vi "setAutoMinMax.vi"(0 "Camera in":refnum<class "Camera.lvclass">, 5 "data_format":T1(ring)=enum."Mono16", 7 "image":u16[][](array[numeric]), 11 "error in (no error)":errorcluster) -> (4 "Camera out":refnum<class "Camera.lvclass">, 15 "error out":errorcluster)   [LabVIEW 2019, in "Camera.lvclass"]
doc: "Retreive the rec handle.\nThis handle allows direct access to all underlying functions of the pco.recorder."
uses:
  Camera.lvclass
  pco.convert/Convert.lvlib
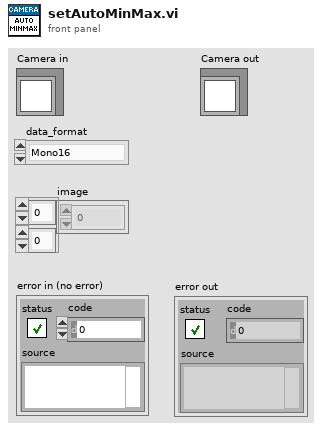
[diagram p1: front panel]
types:
  T1 = enum16{"Undefined", "Mono8", "Mono16", "BGRA8", "RGBA8", "BGRA16", "RGBA16", "CompressedMono8"}
  T2 = cluster{"wScale_minmax":u16, "iScale_maxmax":i32, "iScale_min":i32, "iScale_max":i32, "iColor_temp":i32, "iColor_tint":i32, "iColor_saturation":i32, "iColor_vibrance":i32, "iContrast":i32, "iGamma":i32, "iSRGB":i32, "pHistogramData":u64, "dwProcessingFlags":u32, "wProzValue4Min":u16, "wProzValue4Max":u16}
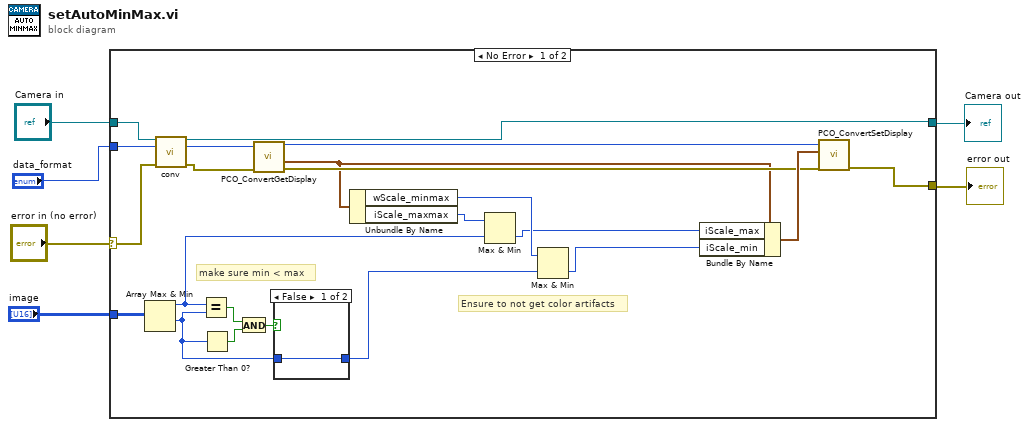
[diagram p0: block diagram]
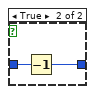
[diagram p2: hidden frame]
diagram:
  n1 = case shown="No Error" "error in (no error)" {
    selector: "error in (no error)" -> [w27 w33]
    tunnel: [w15 w33] -> w4
    tunnel: [w16 w32] -> w5
    tunnel: "Camera in" -> [w28 w32]
    tunnel: "image" -> [w24 _]
    tunnel: "data_format" -> [w14 _]
    frame No Error {
      # "Ensure to not get color artifacts"
      # "make sure min < max"
      n2 = Array Max & Min(array=w24) -> (max value=w12:u16, min value=w20:u16)  [unwired: 2 out]
      n3 = call-dynamic "conv.vi"("Camera in"=w28, "data_format"=w14, "error in (no error)"=w27) -> ("Camera out"=w16:refnum<class "Camera.lvclass">, "conv"=w26:u64, "error out"=w25:errorcluster)  [unwired: 10 in]
      n4 = Equal?(x=w12, y=w20) -> (x = y?=w22:bool)
      n5 = Greater Than 0?(x=w20) -> (x > 0?=w23:bool)
      n6 = And(x=w22, y=w23) -> (x .and. y?=w21:bool)
      n7 = call "PCO_ConvertGetDisplay.vi"("error in (no error)"=w25, "ph"=w26) -> ("error out"=w17:errorcluster, "strDisplay"=w13:T2, "ph out"=w19:u64)  [unwired: 6 in, 1 out]
      n8 = case shown="False" w21 {
        tunnel: w20 -> [w29 w31]
        tunnel: [w29 w30] -> w9
        frame False {
        }
        frame True {
          n9 = Decrement(x=w31) -> (x-1=w30:u16)
        }
      }
      n10 = Unbundle By Name(w13) -> ("wScale_minmax"=w10:u16, "iScale_maxmax"=w11:i32)
      n11 = Max & Min(x=w11, y=w12) -> (min(x,y)=w8:i32)  [unwired: 1 out]
      n12 = Max & Min(x=w10, y=w9) -> (min(x,y)=w7:u16)  [unwired: 1 out]
      n13 = Bundle By Name(cluster=w13, "iScale_max"=w8, "iScale_min"=w7) -> (w18:T2)
      n14 = call "PCO_ConvertSetDisplay.vi"("error in (no error)"=w17, "strDisplay"=w18, "ph"=w19) -> ("error out"=w15:errorcluster)  [unwired: 6 in, 2 out]
    }
    frame Error {
    }
  }
  "error out" <- w4
  "Camera out" <- w5
